vi "Test.vi"   [LabVIEW 2012]
doc: "This VI is called when test mode begins, and will automatically be terminated when it ends. You can add manual or automatic tests and invoke them from the dashboard."
uses:
  <vilib>/Rock Robotics/Network Tables/NT Read Name Cache.vi
  Robot Global Data.vi
  <vilib>/Rock Robotics/Network Tables/NT Globals.vi
  <vilib>/Rock Robotics/Network Tables/Field Data Manager.vi
  <vilib>/Rock Robotics/Network Tables/Table Manager.vi
  <vilib>/Rock Robotics/Network Tables/Report Read Error.vi
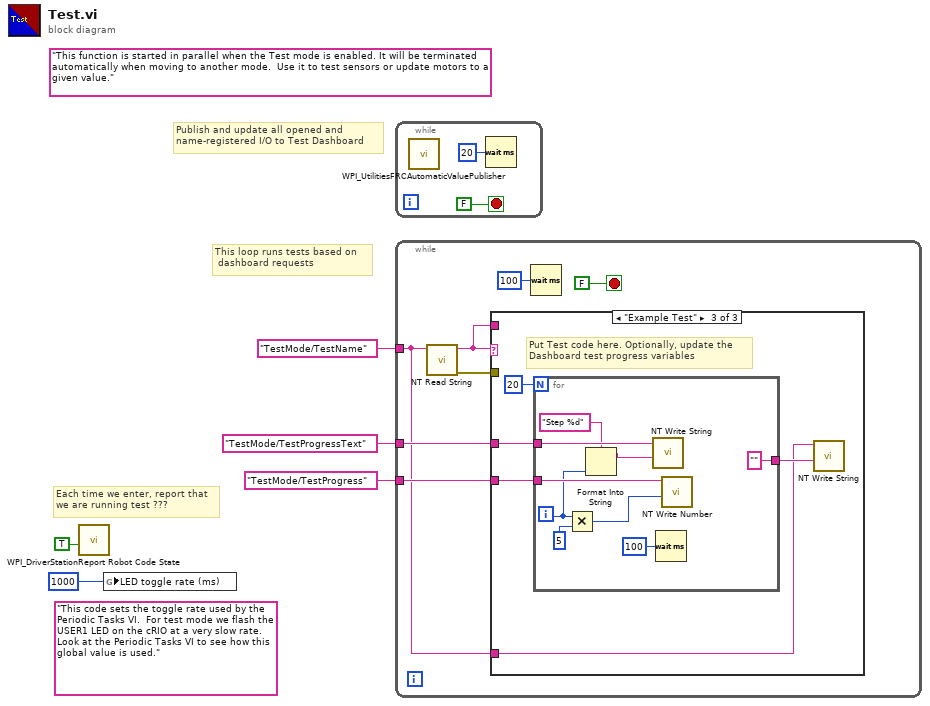
[diagram p0: block diagram]
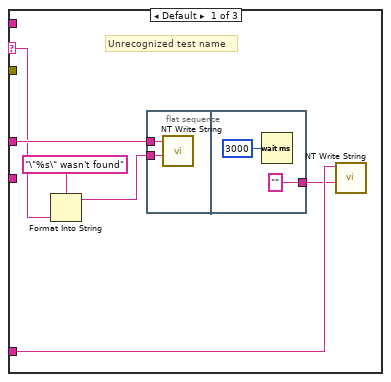
[diagram p2: hidden frame]
diagram:
  (unwired) "This code sets the toggle rate used by the Periodic Tasks VI.  For test mode we flash the USER1 LED on the cRIO at a very slow rate.  Look at the Periodic Tasks VI to see how this global value is used."
  (unwired) "This function is started in parallel when the Test mode is enabled. It will be terminated automatically when moving to another mode.  Use it to test sensors or update motors to a given value."
  # "This loop runs tests based on \n dashboard requests"
  # "Publish and update all opened and\nname-registered I/O to Test Dashboard"
  # "Each time we enter, report that\nwe are running test ???"
  n1 = call <vilib>:"WPI_DriverStationReport Robot Code State.vi"("TeleOp"=TRUE ("Autonomous")) -> ()  [unwired: 10 in, 1 out]
  n2 = global write "Robot Global Data.vi" "LED toggle rate (ms)"(u32 1000 ("LED ms toggle rate")) -> ()
  n3 = while {
    stop <- FALSE stop-if-true
    n4 = call <vilib>:"WPI_UtilitiesFRCAutomaticValuePublisher.vi"() -> ()  [unwired: 12 in]
    n5 = Wait (ms)(milliseconds to wait=u32 20) -> ()  [unwired: 1 out]
  }
  n6 = while {
    tunnel: "TestMode/TestName" ("Name") -> [w9]
    tunnel: "TestMode/TestProgressText" ("Name") -> [w12]
    tunnel: "TestMode/TestProgress" ("Name") -> [w11]
    stop <- FALSE stop-if-true
    n7 = call <vilib>:"NT Read String.vi"("Name"=w9) -> ("error out"=w8:errorcluster, "String"=w10:string)  [unwired: 9 in]
    n8 = case shown="\"Example Test\"" w10 {
      selector: w10 -> [w19 _ _]
      tunnel: w9 -> [w16 _ w25]
      tunnel: w12 -> [w20 _ w28]
      tunnel: w11 -> [_ _ w29]
      tunnel: w10 -> [_ _ _]
      tunnel: w8 -> [_ _ _]
      frame Default {
        # "Unrecognized test name"
        n9 = Format Into String(format string="\"%s\" wasn't found" ("Name"), w19) -> (resulting string=w18:string)  [unwired: 2 in, 1 out]
        n10 = flat-sequence {
          tunnel: w20 -> [w21]
          tunnel: w18 -> [w22]
          tunnel: ["" ("Name")] -> w15
          frame #0 {
            n11 = call <vilib>:"NT Write String.vi"("String"=w22, "Name"=w21) -> ()  [unwired: 9 in, 1 out]
          }
          frame #1 {
            n12 = Wait (ms)(milliseconds to wait=u32 3000) -> ()  [unwired: 1 out]
          }
        }
        n13 = call <vilib>:"NT Write String.vi"("String"=w15, "Name"=w16) -> ()  [unwired: 9 in, 1 out]
      }
      frame "" {
        # "No test to run"
      }
      frame "Example Test" {
        # "Put Test code here. Optionally, update the\nDashboard test progress variables"
        n14 = for {
          N: 20 -> [_]
          tunnel: w29 -> [w38]
          tunnel: w28 -> [w36]
          tunnel: ["" ("String")] -> w26
          i -> [w33]
          n15 = Multiply(x=w33, y=u32 5 ("milliseconds to wait")) -> (x*y=w34:u32)
          n16 = Format Into String(format string="Step %d", w33) -> (resulting string=w31:string)  [unwired: 2 in, 1 out]
          n17 = call <vilib>:"NT Write String.vi"("String"=w31, "Name"=w36) -> ()  [unwired: 9 in, 1 out]
          n18 = Wait (ms)(milliseconds to wait=u32 100) -> ()  [unwired: 1 out]
          n19 = call <vilib>:"NT Write Number.vi"("Numeric"=w34, "Name"=w38) -> ()  [unwired: 9 in, 1 out]
        }
        n20 = call <vilib>:"NT Write String.vi"("String"=w26, "Name"=w25) -> ()  [unwired: 9 in, 1 out]
      }
    }
    n21 = Wait (ms)(milliseconds to wait=u32 100) -> ()  [unwired: 1 out]
  }
